vi "GetLinkerDependencyFromFiles.vi"(9 "Overwrite LabVIEW Folder(If empty use this version of LabVIEW)":path, 11 "All Files in Dir":path[](array[path])) -> (3 "FileDependency":map{path, T1}(c390))   [LabVIEW 2020, in "DependencyChecker.lvlib"]
uses:
  DependencyChecker.lvlib
  FileDependencyType.ctl
  <vilib>/Utility/lvfile.llb/FT_FileTypes.ctl
  fa84a50a-7a91-41f1-93a7-6c8b41b91fd3.vi
  <vilib>/Utility/lvfile.llb/NI_FileType.lvlib
panel:
  in  "x":path
  out "Dependecy":T1
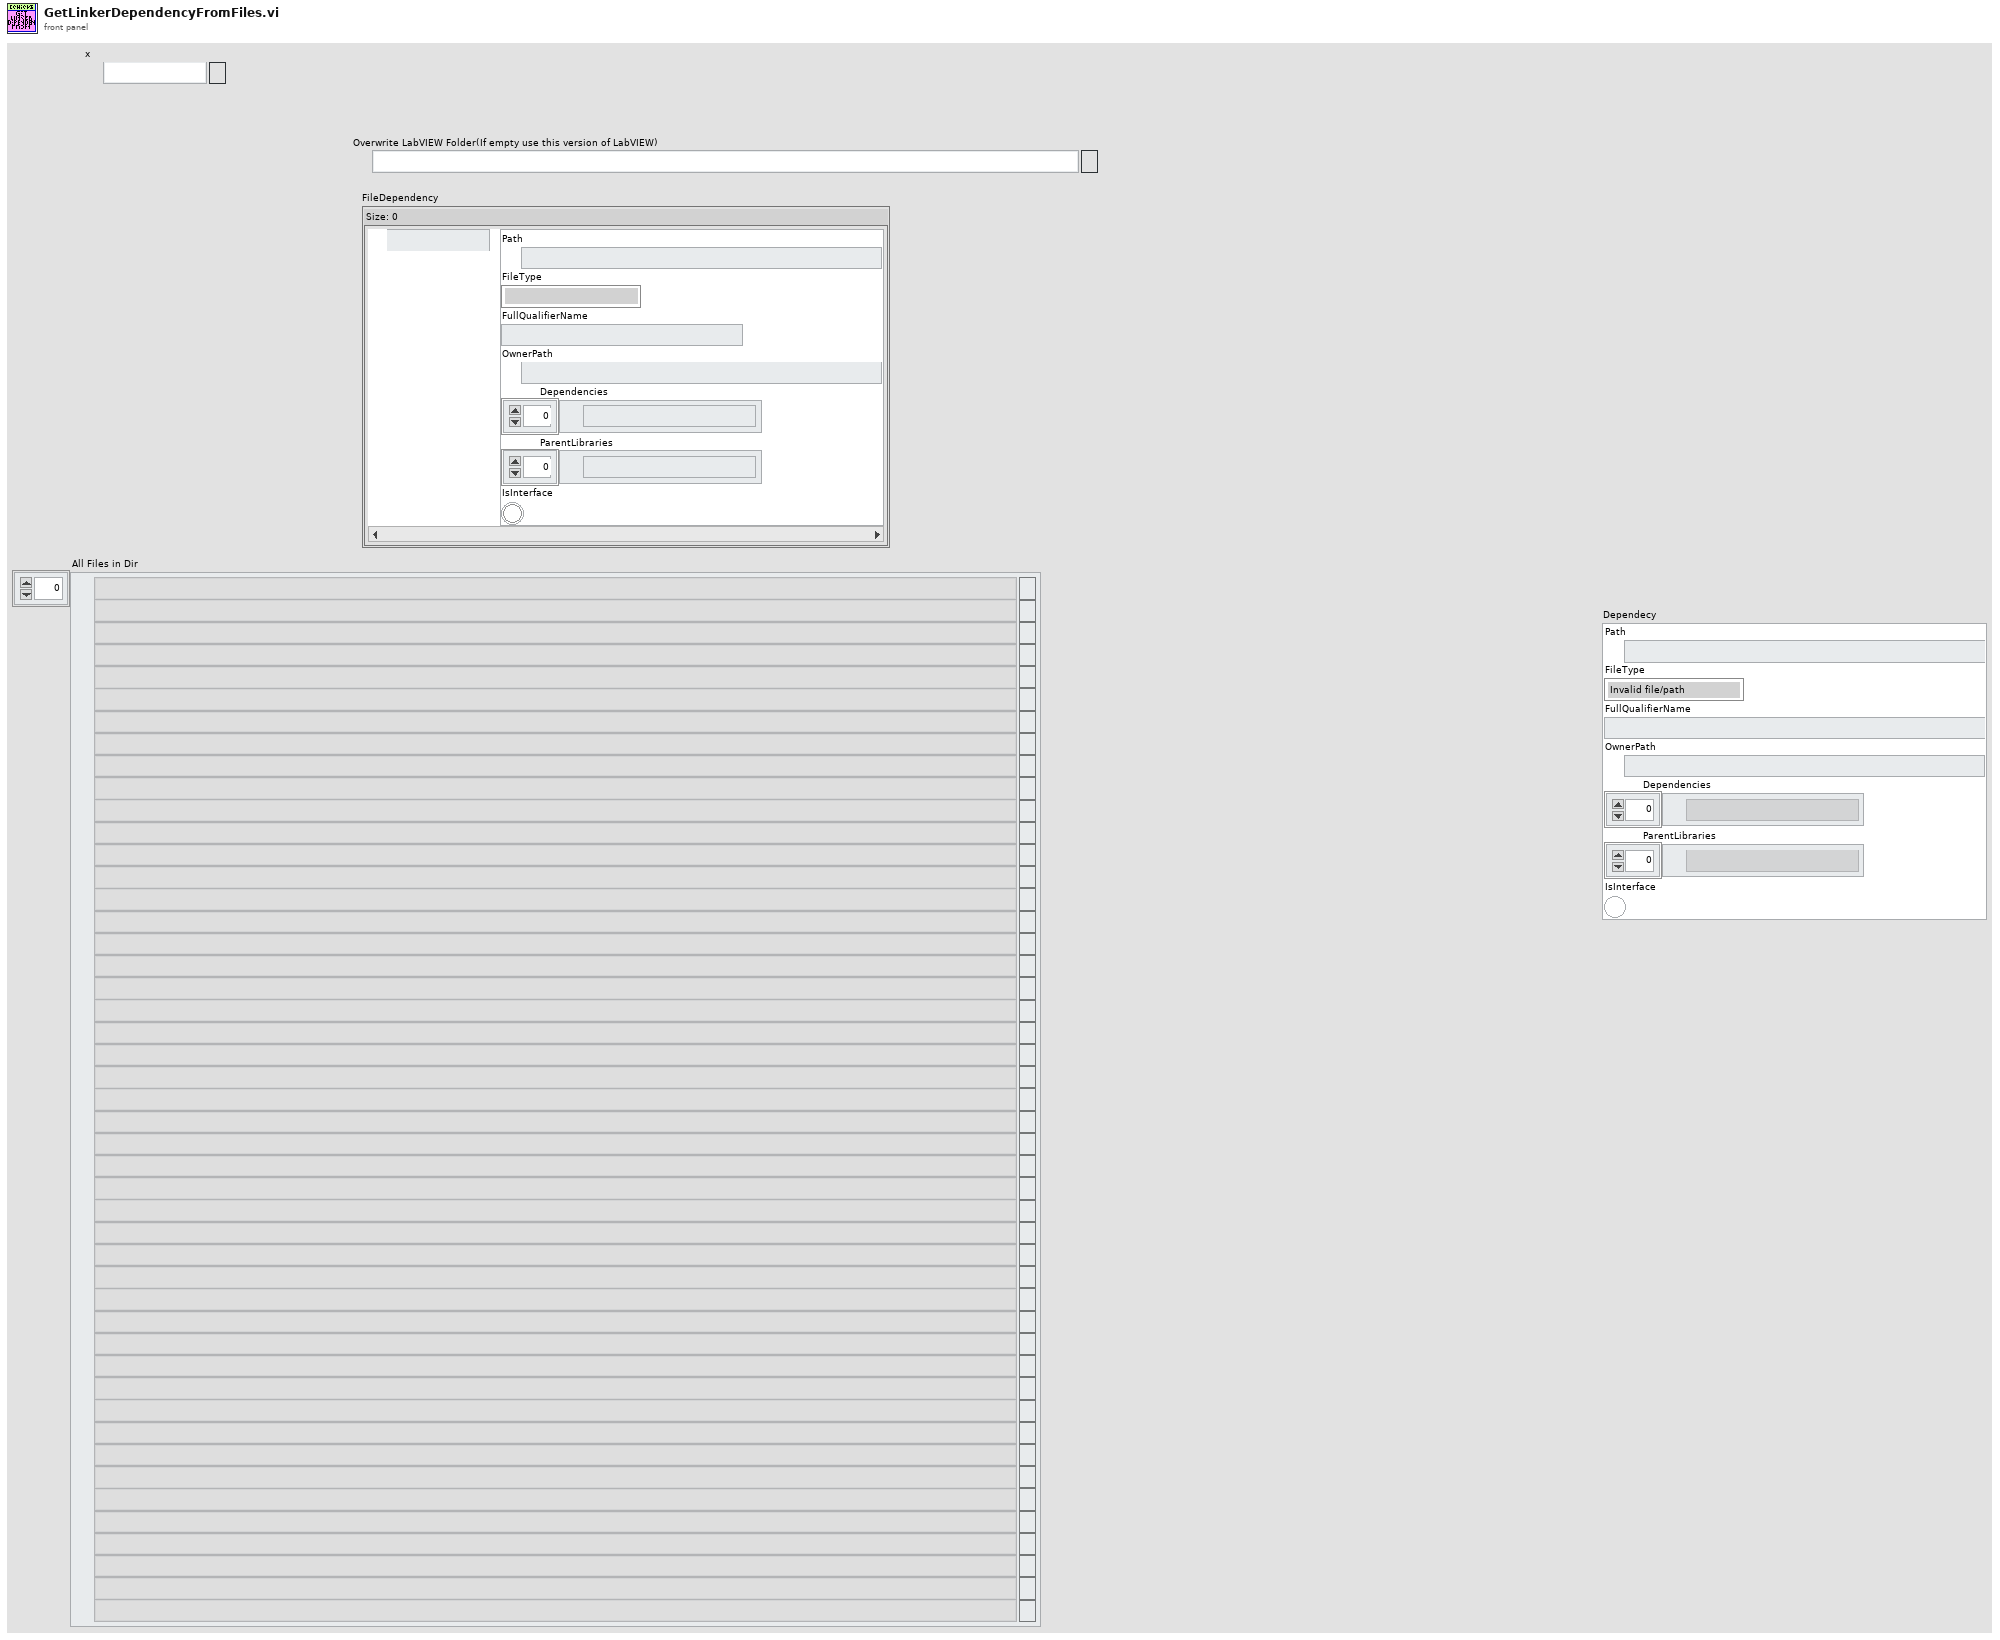
[diagram p1: front panel]
types:
  T1 = typedef "DependencyChecker.lvlib/FileDependencyType.ctl" = cluster{"Path":path, "FileType":T2, "FullQualifierName":string, "OwnerPath":path, "Dependencies":path[], "ParentLibraries":path[], "IsInterface":bool}
  T2 = typedef "NI_FileType.lvlib/FT_FileTypes.ctl" = enum32{"Invalid file/path", "Unknown type", "Instrument", "Control", "Polymorphic VI", "Project", "Library", "LVClass", "XControl", "XNode", "CIN", "Run-time menu", "Palette menu", "LLB", "Shortcut", "Directory", "Class Private Data Control", "Statechart", "MathScript .m file", "Ladder Diagram", "LVLibp"}
  T3 = typedef "NI_FileType.lvlib/LVFileType.ctl" = enum32{"Invalid file", "Unknown type", "Instrument", "Control", "Polymorphic VI", "Project", "Library", "LVClass", "XControl", "XNode", "Shared library", ".NET assembly", "ActiveX interface", "CIN", "Run-time menu", "Palette menu", "Help file", "LLB", "XNode Edit Dependency", "Class Private Data Control", "Statechart", "MathScript .m file", "Ladder Diagram", "LVLibp", "XNode Build Dependency"}
  T4 = cluster{"path":path, "delimited name":string, "type":T3, "iState":u32, "iStyle":u16, "wStyle":u16, "buttons":u16, "viflags":u32, "viflags2":u32, "links":u32[]}[]
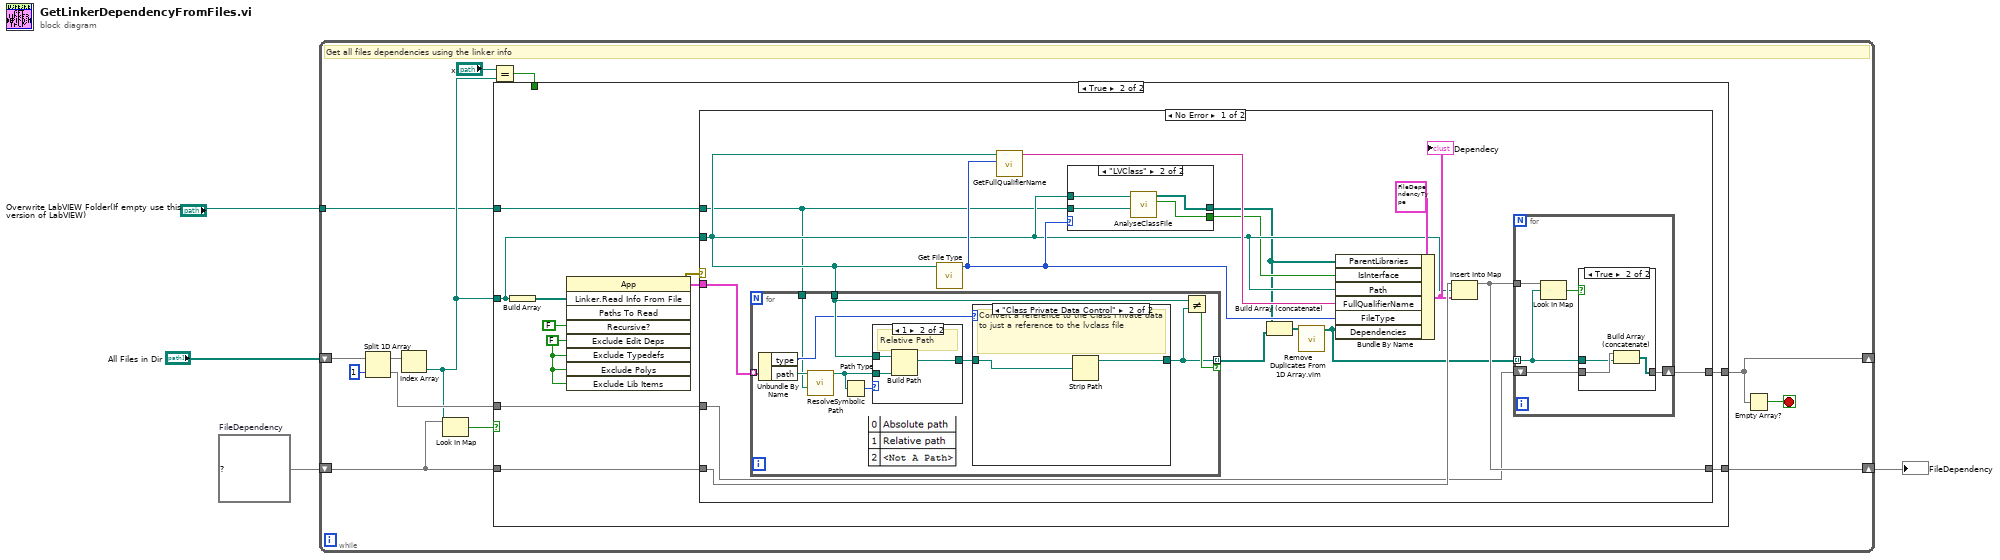
[diagram p0: block diagram]
diagram:
  w3 = map{path, T1} {}  # FileDependency
  n1 = while {
    shift-right: [w13] -> w4
    shift-left: w3 -> [w10]
    shift-right: [w11] -> _
    shift-left: "All Files in Dir" -> [w17]
    tunnel: "Overwrite LabVIEW Folder(If empty use this version of LabVIEW)" -> [w5]
    stop <- w12 stop-if-true
    # "Get all files dependencies using the linker info"
    n2 = Split 1D Array(array=w17, index=1) -> (first subarray=w15:path[], second subarray=w14:path[])
    n3 = Index Array(array=w15) -> (element=w8:path)  [unwired: 1 in]
    n4 = Look In Map(map=w10, key=w8) -> (key not found?=w9:bool)  [unwired: 1 in, 1 out]
    n5 = Equal?(x="x", y=w8) -> (x = y?=w6:bool)
    n6 = case shown="True" w9 {
      tunnel: w14 -> [w18 w30]
      tunnel: [w19 w29] -> w13
      tunnel: [w18 w28] -> w11
      tunnel: w10 -> [w19 w23]
      tunnel: w8 -> [_ w22]
      tunnel: w6 -> [_ _]
      tunnel: w5 -> [_ w20]
      frame False {
      }
      frame True {
        w21 = FALSE ("Exclude Edit Time Dependencies")
        n7 = Build Array(w22) -> (w27:path[])
        n8 = invoke class="App" method="Linker.Read Info From File"("Paths To Read"=w27, "Recursive?"=FALSE, "Exclude Edit Deps"=w21, "Exclude Typedefs"=w21, "Exclude Polys"=w21, "Exclude Lib Items"=w21) -> (error out=w24:errorcluster, "Linker.Read Info From File"=w25:T4)  [unwired: 3 in, 7 out]
        n9 = case shown="No Error" w24 {
          tunnel: w25 -> [w45 _]
          tunnel: w23 -> [w46 w77]
          tunnel: w30 -> [w42 w78]
          tunnel: [w41 w78] -> w28
          tunnel: w22 -> [w36 _]
          tunnel: [w43 w77] -> w29
          tunnel: w20 -> [w31 _]
          frame No Error {
            n10 = for {
              tunnel: w45 -> [w69] mode=indexing
              tunnel: [w61] -> w37 mode=indexing if=w66
              tunnel: w36 -> [w65]
              tunnel: w31 -> [w60]
              n11 = Unbundle By Name(w69) -> ("type"=w63:T3, "path"=w67:path)
              n12 = call "ResolveSymbolicPath.vi"("Overwrite LabVIEW Folder(If empty use this version of LabVIEW)"=w60, "path"=w67) -> ("File Path"=w64:path)  [unwired: 9 in]
              n13 = Path Type(1:w64) -> (0:w68:i16)
              n14 = case shown="1" w68 {
                tunnel: w64 -> [w73 w76]
                tunnel: [w73 w74] -> w62
                tunnel: w65 -> [_ w75]
                frame 0, Default {
                  # "Absolute Path"
                }
                frame 1 {
                  # "Relative Path"
                  n15 = Build Path(base path=w75, name or relative path=w76) -> (appended path=w74:path)
                }
              }
              n16 = case shown="\"Class Private Data Control\"" w63 {
                tunnel: w62 -> [w70 w72]
                tunnel: [w70 w71] -> w61
                frame Default {
                }
                frame "Class Private Data Control" {
                  # "Convert a reference to the Class Private data to just a reference to the lvclass file"
                  n17 = Strip Path(path=w72) -> (stripped path=w71:path)  [unwired: 1 out]
                }
              }
              n18 = Not Equal?(x=w65, y=w61) -> (x != y?=w66:bool)
            }
            n19 = call <vilib>:"Get File Type.vi"("path"=w36) -> ("file type"=w39:T2)  [unwired: 8 in, 2 out]
            n20 = call "GetFullQualifierName.vi"("file type"=w39, "File Path"=w36) -> ("FullQualifierName"=w40:string)  [unwired: 9 in]
            n21 = case shown="\"LVClass\"" w39 {
              tunnel: w36 -> [_ w50]
              tunnel: [_ w49] -> w34
              tunnel: [_ w48] -> w35
              tunnel: w31 -> [_ w47]
              frame "Invalid file/path", Default {
              }
              frame "LVClass" {
                n22 = call "AnalyseClassFile.vi"("Overwrite LabVIEW Folder(If empty use this version of LabVIEW)"=w47, "File Path"=w50) -> ("IsInterface"=w48:bool, "ParentLibraries"=w49:path[])  [unwired: 8 in]
              }
            }
            n23 = Build Array (concatenate)(w34, w37) -> (w33:path[])
            n24 = call "Remove Duplicates From 1D Array.vim"("array"=w33) -> ("array with duplicates removed"=w32:path[])  [unwired: 10 in]
            n25 = Bundle By Name(cluster=T1 {"Path"=path "", "FileType"=enum."Instrument", "FullQualifierName"="Decorator1_Main.vi", "OwnerPath"=path "", "Dependencies"=[], "ParentLibraries"=[], "IsInterface"=FALSE} ("value"), "ParentLibraries"=w34, "IsInterface"=w35, "Path"=w36, "FullQualifierName"=w40, "FileType"=w39, "Dependencies"=w32) -> (w44:T1)
            "Dependecy" <- w44
            n26 = Insert Into Map(map in=w46, key=w36, value=w44) -> (map out=w43:map{path, T1})  [unwired: 2 out]
            n27 = for {
              tunnel: w43 -> [w55]
              tunnel: w32 -> [w51] mode=indexing
              shift-right: [w52] -> w41
              shift-left: w42 -> [w53]
              n28 = Look In Map(map=w55, key=w51) -> (key not found?=w54:bool)  [unwired: 1 in, 1 out]
              n29 = case shown="True" w54 {
                tunnel: w53 -> [w56 w59]
                tunnel: [w56 w58] -> w52
                tunnel: w51 -> [_ w57]
                frame False {
                }
                frame True {
                  n30 = Build Array (concatenate)(w59, w57) -> (w58:path[])
                }
              }
            }
          }
          frame Error {
          }
        }
      }
    }
    n31 = Empty Array?(array=w11) -> (empty?=w12:bool)
  }
  "FileDependency" <- w4
